vi "Write Single Coil.vi"(8 "error in":errorcluster, 9 "coil value":bool, 10 "address":u16, 11 "Master CR in":refnum<class "Master CR.lvclass">) -> (0 "error out":errorcluster, 3 "Master CR out":refnum<class "Master CR.lvclass">)   [LabVIEW 2021, in "Master CR.lvclass"]
doc: "Writes the value of a single coil."
uses:
  Master CR.lvclass
  Master CR.lvclass/Master CR.ctl
  Modbus_v121c/Data Model/Device Data Model.lvclass
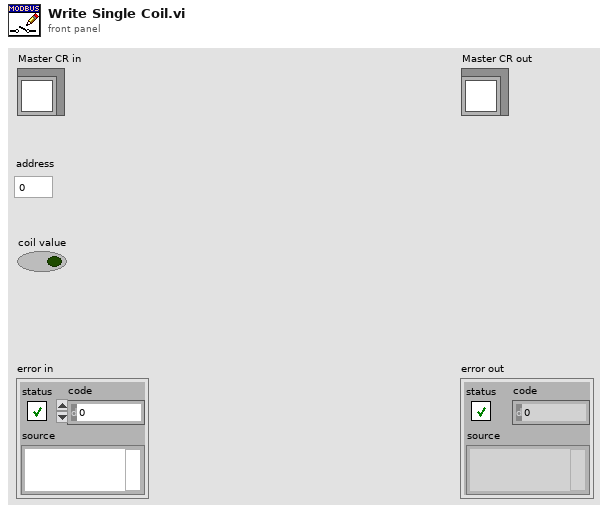
[diagram p1: front panel]
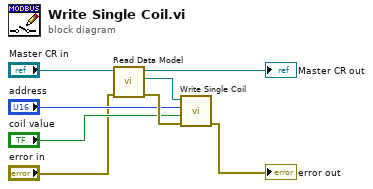
[diagram p0: block diagram]
diagram:
  n1 = call "Read Data Model.vi"("error in (no error)"="error in", "Master CR in"="Master CR in") -> ("error out"=w5:errorcluster, "Data Model"=w8:refnum<class "Device Data Model.lvclass">, "Master CR out"=→"Master CR out":refnum<class "Master CR.lvclass">)  [unwired: 7 in]
  n2 = call-dynamic "Write Single Coil.vi"("error in"=w5, "coil value"="coil value", "address"="address", "device data model in"=w8) -> ("error out"=→"error out":errorcluster)  [unwired: 6 in, 1 out]
